vi "Machs2-15-07-2017.vi"(0 "d0Mach1":fxp<+/-,18,18> format="%.16g", 1 "heizenMach1":bool, 2 "U_SPMach1":fxp<+/-,26,5> format="%.23g", 3 "->Register":u32, 5 "d1Mach1":fxp<+/-,21,21> format="%.16g", 7 "Warten(uSec)":u16=5000, 9 "d0Mach2":fxp<+/-,18,18> format="%.16g", 11 "d1Mach2":fxp<+/-,21,21> format="%.16g", 12 "heizenMach2":bool, 13 "U_SPMach2":fxp<+/-,26,5> format="%.23g") -> (4 "U_MWMach1":fxp<+/-,26,5> format="%.23g", 14 "Register->":u32, 15 "U_MWMach2":fxp<+/-,26,5> format="%.23g")   [LabVIEW 2010]
uses:
  <vilib>/eio/EIONode/EIONode.xnode
  <vilib>/rvi/eio/nirviEIOImplementation/nirviEIOImplementation.xnode
  <vilib>/rvi/eio/common/nirviEmuClasses.ctl
  <vilib>/rvi/FXPMathLib/FxpAdd/XNode/nifxpmath_Add.xnode
  <vilib>/rvi/FXPMathLib/FxpAdd/subVIs/nifxpmath_Add_SimConfig.ctl
  <vilib>/fxp/LVFixedPointQuantizationPolicyTypeDef.ctl
  <vilib>/fxp/LVFixedPointOverflowPolicyTypeDef.ctl
  <vilib>/rvi/FXPMathLib/FxpDiv/XNode/nifxpmath_Div.xnode
  <vilib>/rvi/FXPMathLib/FxpDiv/subVIs/nifxpmath_Div_SimConfig.ctl
  <vilib>/rvi/FXPMathLib/FxpMul/XNode/nifxpmath_Multiplier.xnode
  <vilib>/rvi/FXPMathLib/FxpMul/subVIs/nifxpmath_Mul_SimConfig.ctl
  <vilib>/rvi/FXPMathLib/FxpSqrt/XNode/nifxpmath_Sqrt.xnode
  <vilib>/rvi/FXPMathLib/FxpSqrt/subVIs/nifxpmath_Sqrt_SimConfig.ctl
  <vilib>/rvi/FXPMathLib/FxpConvert/XNode/nifxpmath_Convert.xnode
  <vilib>/rvi/FXPMathLib/FxpConvert/subVIs/nifxpmath_Convert_SimConfig.ctl
  <vilib>/rvi/FXPMathLib/FxpSub/XNode/nifxpmath_Sub.xnode
  <vilib>/rvi/FXPMathLib/FxpSub/subVIs/nifxpmath_Sub_SimConfig.ctl
  <vilib>/rvi/eio/common/nirviEmuTemplateMethod_noerrors.vi
  <vilib>/rvi/FXPMathLib/FxpAdd/simVIs/DllFxpAddTemp_sub.vi
  <vilib>/rvi/FXPMathLib/FxpDiv/simVIs/DllFxpDivTemp_sub.vi
  <vilib>/rvi/FXPMathLib/FxpMul/simVIs/DllFxpMulTemp_sub.vi
  <vilib>/rvi/FXPMathLib/FxpSqrt/simVIs/DllSqrtTemp_sub.vi
  <vilib>/rvi/FXPMathLib/FxpConvert/simVIs/DllFxpConvertTemp_sub.vi
  <vilib>/rvi/FXPMathLib/FxpSub/simVIs/DllFxpSubTemp_sub.vi
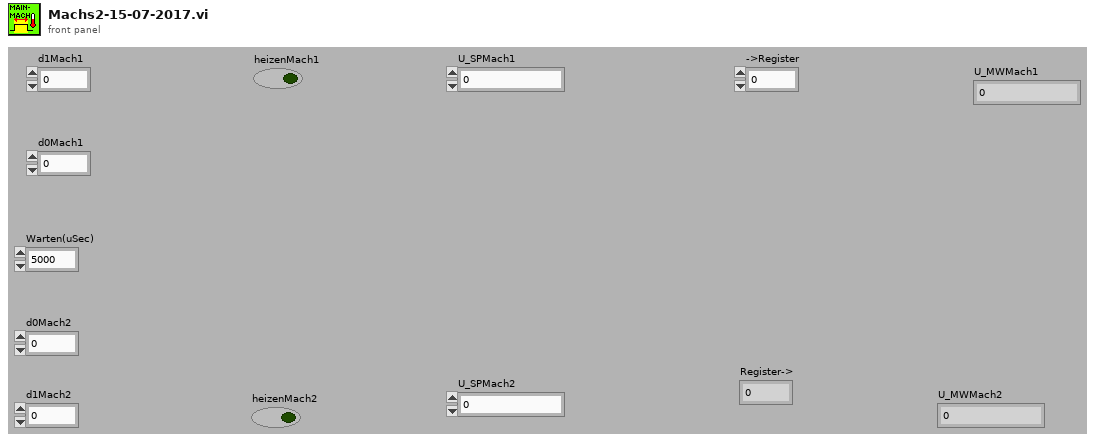
[diagram p1: front panel]
types:
  T1 = typedef "nirviEmuClasses.ctl" = enum16{"IO Read", "IO Write", "Method", "Property Read", "Property Write"}
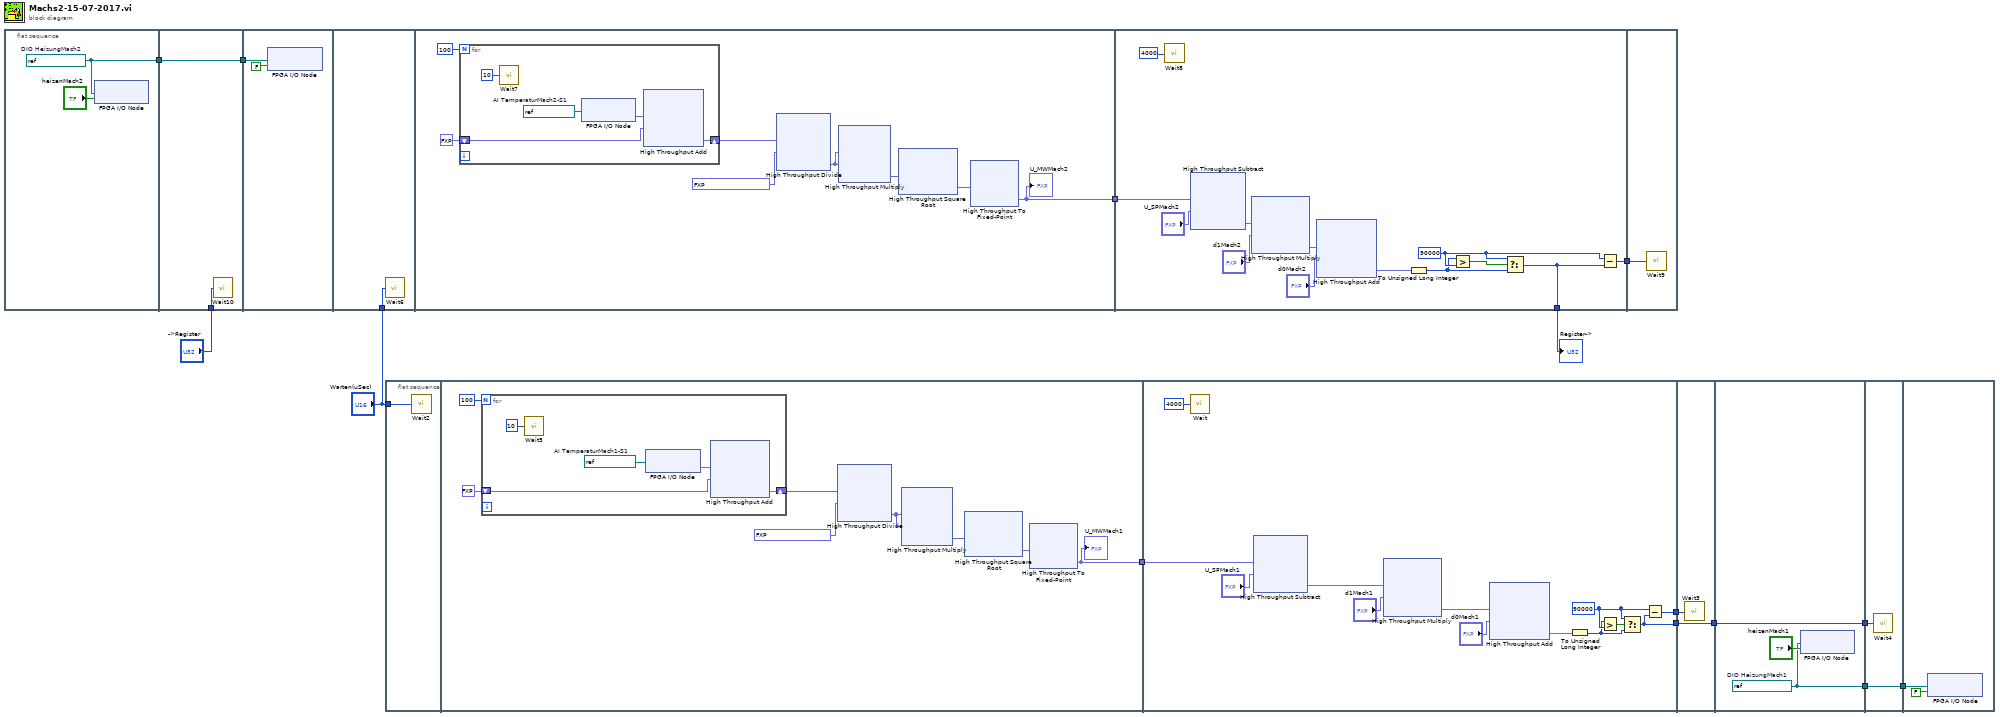
[diagram p0: block diagram]
diagram:
  n1 = flat-sequence {
    tunnel: [w15] -> w1
    tunnel: "->Register" -> [w29]
    tunnel: [w28] -> w2
    tunnel: w1 -> [w28]
    tunnel: w2 -> [w30]
    tunnel: "Warten(uSec)" -> [w43]
    tunnel: [w44] -> w8
    tunnel: w8 -> [w217]
    tunnel: [w211] -> w7
    tunnel: [w207] -> w6
    tunnel: w7 -> [w307]
    frame #0 {
      w15 = refnum<k21> "Mod6/DIO17"  # DIO HeizungMach2
      n2 = xnode "FPGA I/O Node"("I/O Item"="heizenMach2", "FPGA I/O In"=w15) -> ()  [unwired: 1 out]
    }
    frame #1 {
      n3 = call "Wait10"("Count(uSec)"=w29) -> ()  [unwired: 1 out]
    }
    frame #2 {
      n4 = xnode "FPGA I/O Node"("I/O Item"=FALSE, "FPGA I/O In"=w30) -> ()  [unwired: 1 out]
    }
    frame #3 {
      n5 = call "Wait6"("Count(uSec)"=w43) -> ()  [unwired: 1 out]
    }
    frame #4 {
      n6 = for {
        N: 100 -> [_]
        shift-right: [w154] -> w51
        shift-left: fxp<+/-,33,12> 0.0 ("x+y") -> [w155]
        w153 = refnum<k21> "Mod1/AI7"  # AI TemperaturMach2-S1
        n7 = call "Wait7"("Count(uSec)"=u8 10) -> ()  [unwired: 1 out]
        n8 = xnode "FPGA I/O Node"("FPGA I/O In"=w153) -> ("I/O Item"=w156:fxp<+/-,26,5>)  [unwired: 1 out]
        n9 = xnode "High Throughput Add"("x"=w156, "y"=w155) -> ("x+y"=w154:fxp<+/-,33,12>)
      }
      n10 = xnode "High Throughput Divide"("x"=w51, "y"=fxp<+/-,8,8> 100.0) -> ("x/y"=w47:fxp<+/-,26,5>)
      n11 = xnode "High Throughput Multiply"("x"=w47, "y"=w47) -> ("x*y"=w46:fxp<+,52,10>)
      n12 = xnode "High Throughput Square Root"("x"=w46) -> ("sqrt(x)"=w45:fxp<+,26,5>)
      n13 = xnode "High Throughput To Fixed-Point"("x"=w45) -> ("y"=w44:fxp<+/-,26,5>)
      "U_MWMach2" <- w44
    }
    frame #5 {
      w209 = u32 90000 ("x")
      n14 = call "Wait8"("Count(uSec)"=u16 4000) -> ()  [unwired: 1 out]
      n15 = xnode "High Throughput Subtract"("x"=w217, "y"="U_SPMach2") -> ("x-y"=w216:fxp<+/-,26,5>)
      n16 = xnode "High Throughput Multiply"("x"=w216, "y"="d1Mach2") -> ("x*y"=w214:fxp<+/-,18,18>)
      n17 = xnode "High Throughput Add"("x"=w214, "y"="d0Mach2") -> ("x+y"=w212:fxp<+/-,18,18>)
      n18 = To Unsigned Long Integer(number=w212) -> (unsigned 32bit integer=w208:u32)
      n19 = Greater?(x=w208, y=w209) -> (0:w210:bool)
      n20 = Select(t=w209, s=w210, f=w208) -> (s? t:f=w207:u32)
      n21 = Subtract(x=w209, y=w207) -> (x-y=w211:u32)
    }
    frame #6 {
      n22 = call "Wait9"("Count(uSec)"=w307) -> ()  [unwired: 1 out]
    }
  }
  n23 = flat-sequence {
    tunnel: "Warten(uSec)" -> [w308]
    tunnel: [w309] -> w13
    tunnel: w13 -> [w482]
    tunnel: [w472] -> w12
    tunnel: [w476] -> w11
    tunnel: [w573] -> w10
    tunnel: w12 -> [w573]
    tunnel: w11 -> [w572]
    tunnel: [w575] -> w9
    tunnel: w10 -> [w575]
    tunnel: [w574] -> w3
    tunnel: w9 -> [w589]
    tunnel: [w588] -> w4
    tunnel: w3 -> [w588]
    tunnel: w4 -> [w590]
    frame #0 {
      n24 = call "Wait2"("Count(uSec)"=w308) -> ()  [unwired: 1 out]
    }
    frame #1 {
      n25 = for {
        N: 100 -> [_]
        shift-right: [w419] -> w316
        shift-left: fxp<+/-,33,12> 0.0 ("x+y") -> [w420]
        w418 = refnum<k21> "Mod1/AI5"  # AI TemperaturMach1-S1
        n26 = call "Wait5"("Count(uSec)"=u8 10) -> ()  [unwired: 1 out]
        n27 = xnode "FPGA I/O Node"("FPGA I/O In"=w418) -> ("I/O Item"=w421:fxp<+/-,26,5>)  [unwired: 1 out]
        n28 = xnode "High Throughput Add"("x"=w421, "y"=w420) -> ("x+y"=w419:fxp<+/-,33,12>)
      }
      n29 = xnode "High Throughput Divide"("x"=w316, "y"=fxp<+/-,8,8> 100.0) -> ("x/y"=w312:fxp<+/-,26,5>)
      n30 = xnode "High Throughput Multiply"("x"=w312, "y"=w312) -> ("x*y"=w311:fxp<+,52,10>)
      n31 = xnode "High Throughput Square Root"("x"=w311) -> ("sqrt(x)"=w310:fxp<+,26,5>)
      n32 = xnode "High Throughput To Fixed-Point"("x"=w310) -> ("y"=w309:fxp<+/-,26,5>)
      "U_MWMach1" <- w309
    }
    frame #2 {
      w474 = u32 90000 ("x")
      n33 = call "Wait"("Count(uSec)"=u16 4000) -> ()  [unwired: 1 out]
      n34 = xnode "High Throughput Subtract"("x"=w482, "y"="U_SPMach1") -> ("x-y"=w481:fxp<+/-,26,5>)
      n35 = xnode "High Throughput Multiply"("x"=w481, "y"="d1Mach1") -> ("x*y"=w479:fxp<+/-,18,18>)
      n36 = xnode "High Throughput Add"("x"=w479, "y"="d0Mach1") -> ("x+y"=w477:fxp<+/-,18,18>)
      n37 = To Unsigned Long Integer(number=w477) -> (unsigned 32bit integer=w473:u32)
      n38 = Greater?(x=w473, y=w474) -> (0:w475:bool)
      n39 = Select(t=w474, s=w475, f=w473) -> (s? t:f=w472:u32)
      n40 = Subtract(x=w474, y=w472) -> (x-y=w476:u32)
    }
    frame #3 {
      n41 = call "Wait3"("Count(uSec)"=w572) -> ()  [unwired: 1 out]
    }
    frame #4 {
      w574 = refnum<k21> "Mod6/DIO28"  # DIO HeizungMach1
      n42 = xnode "FPGA I/O Node"("I/O Item"="heizenMach1", "FPGA I/O In"=w574) -> ()  [unwired: 1 out]
    }
    frame #5 {
      n43 = call "Wait4"("Count(uSec)"=w589) -> ()  [unwired: 1 out]
    }
    frame #6 {
      n44 = xnode "FPGA I/O Node"("I/O Item"=FALSE, "FPGA I/O In"=w590) -> ()  [unwired: 1 out]
    }
  }
  "Register->" <- w6
